vi "Attenuator_FindZero.vi"(2 "error in (no error)":errorcluster caption="错误输入（无错误）", 3 "Axis":u16) -> (0 "error out":errorcluster caption="错误输出")   [LabVIEW 2018]
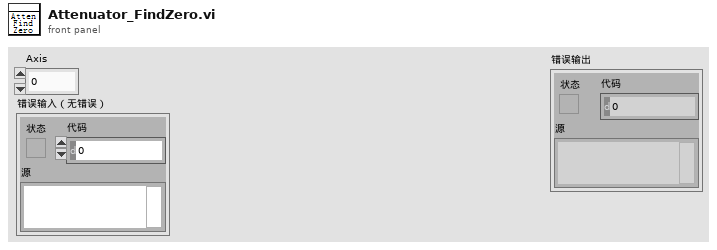
[diagram p1: front panel]
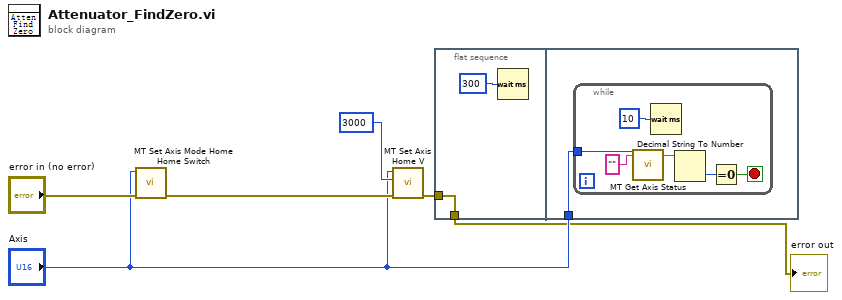
[diagram p0: block diagram]
diagram:
  n1 = call "MT Set Axis Mode Home Home Switch.vi"("error in (no error)"="error in (no error)", "AObj"="Axis") -> ("error out"=w5:errorcluster)  [unwired: 8 in, 1 out]
  n2 = call "MT Set Axis Home V.vi"("error in (no error)"=w5, "Value"=3000, "AObj"="Axis") -> ("error out"=w3:errorcluster)  [unwired: 7 in, 1 out]
  n3 = flat-sequence {
    tunnel: w3 -> [w7]
    tunnel: [w7] -> w1
    tunnel: "Axis" -> [w9]
    frame #0 {
      n4 = Wait (ms)(milliseconds to wait=u32 300 ("等待时间（毫秒）")) -> ()  [unwired: 1 out]
    }
    frame #1 {
      n5 = while {
        tunnel: w9 -> [w15]
        stop <- w11 stop-if-true
        n6 = call "MT Get Axis Status.vi"("AObj"=w15, "pRun"="") -> ("pRun out"=w13:string)  [unwired: 18 in, 7 out]
        n7 = Wait (ms)(milliseconds to wait=u32 10 ("等待时间（毫秒）")) -> ()  [unwired: 1 out]
        n8 = Decimal String To Number(string=w13) -> (number=w12:i32)  [unwired: 2 in, 1 out]
        n9 = Equal To 0?(x=w12) -> (x = 0?=w11:bool)
      }
    }
  }
  "error out" <- w1
